vi "Run.vi"(8 "error in (no error)":errorcluster, 11 "SPARC4_GUI in":refnum<class "S4GEI.lvclass">) -> (0 "error out":errorcluster, 3 "SPARC4_GUI out":refnum<class "S4GEI.lvclass">)   [LabVIEW 2018, in "S4GEI.lvclass"]
uses:
  S4GEI.lvclass
  S4GEI.lvclass/S4GEI.ctl
  Channel GUI/Channel.lvclass
  S4ICS/S4ICS.lvclass
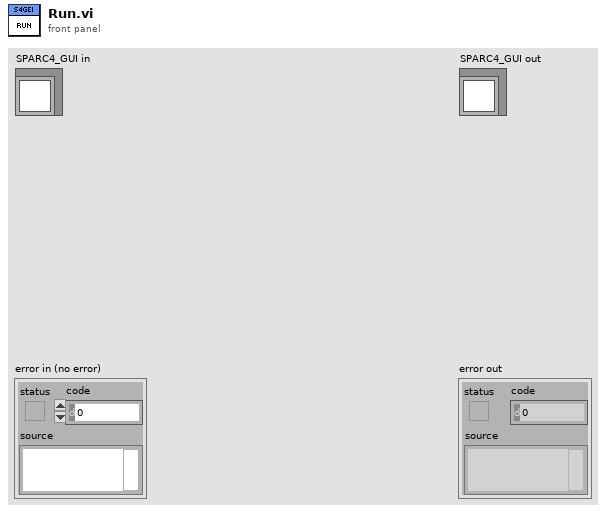
[diagram p1: front panel]
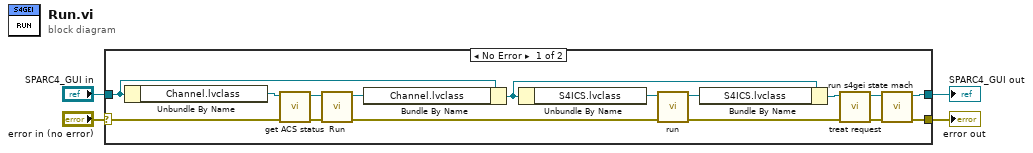
[diagram p0: block diagram]
diagram:
  n1 = case shown="No Error" "error in (no error)" {
    selector: "error in (no error)" -> [w15 w22]
    tunnel: [w9 w22] -> w3
    tunnel: [w10 w21] -> w1
    tunnel: "SPARC4_GUI in" -> [w19 w21]
    frame No Error {
      n2 = Unbundle By Name(w19) -> ("Channel.lvclass"=w18:refnum<class "Channel.lvclass">)
      n3 = call "get ACS status.vi"("error in (no error)"=w15, "Channel in"=w18) -> ("error out"=w16:errorcluster, "Channel out"=w17:refnum<class "Channel.lvclass">)  [unwired: 8 in]
      n4 = call "Run.vi"("error in (no error)"=w16, "Channel GUI in"=w17) -> ("error out"=w11:errorcluster, "Channel GUI out"=w20:refnum<class "Channel.lvclass">)  [unwired: 8 in]
      n5 = Bundle By Name(cluster=w19, "Channel.lvclass"=w20) -> (w13:refnum<class "S4GEI.lvclass">)
      n6 = Unbundle By Name(w13) -> ("S4ICS.lvclass"=w14:refnum<class "S4ICS.lvclass">)
      n7 = call "run.vi"("error in (no error)"=w11, "S4ICS in"=w14) -> ("error out"=w5:errorcluster, "S4ICS out"=w12:refnum<class "S4ICS.lvclass">)  [unwired: 8 in]
      n8 = Bundle By Name(cluster=w13, "S4ICS.lvclass"=w12) -> (w8:refnum<class "S4GEI.lvclass">)
      n9 = call "treat request.vi"("error in (no error)"=w5, "S4GEI in"=w8) -> ("error out"=w6:errorcluster, "S4GEI out"=w7:refnum<class "S4GEI.lvclass">)  [unwired: 8 in]
      n10 = call "run s4gei state mach.vi"("error in (no error)"=w6, "S4GEI in"=w7) -> ("error out"=w9:errorcluster, "S4GEI out"=w10:refnum<class "S4GEI.lvclass">)  [unwired: 8 in]
    }
    frame Error {
    }
  }
  "error out" <- w3
  "SPARC4_GUI out" <- w1
